vi "zmq_socket_set.vi"(7 "dll":path, 8 "error in":errorcluster, 10 "socket":u64, 11 "context":u64) -> (0 "error out":errorcluster, 3 "socket out":refnum<class "Socket.lvclass">)   [LabVIEW 2025, in "ZeroMQ.lvlib" / "Socket.lvclass"]
uses:
  Socket.lvclass
  Socket.lvclass/Socket.ctl
panel:
  # "ØMQ"
  # "labview"
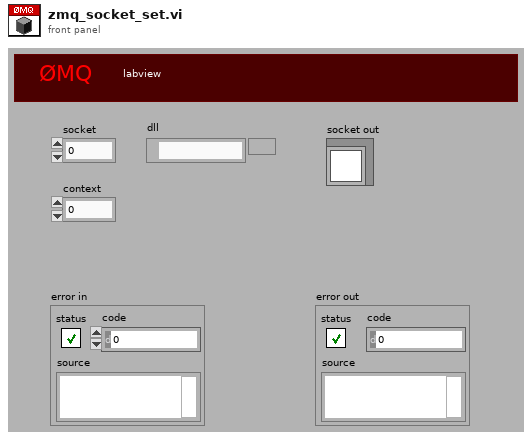
[diagram p1: front panel]
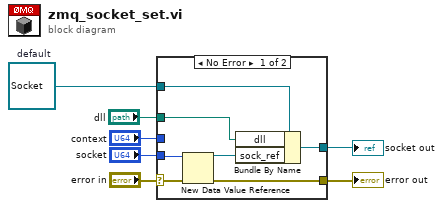
[diagram p0: block diagram]
diagram:
  w7 = refnum<class "Socket.lvclass"> refnum  # default
  n1 = case shown="No Error" "error in" {
    selector: "error in" -> [w9 w15]
    tunnel: w7 -> [w14 _]
    tunnel: [w13 _] -> w6
    tunnel: [w10 w15] -> w4
    tunnel: "context" -> [_ _]
    tunnel: "socket" -> [w11 _]
    tunnel: "dll" -> [w8 _]
    frame No Error {
      n2 = New Data Value Reference(data value=w11, error in=w9) -> (data value reference=w12:refnum<data-value>, error out=w10:errorcluster)
      n3 = Bundle By Name(cluster=w14, "dll"=w8, "sock_ref"=w12) -> (w13:refnum<class "Socket.lvclass">)
    }
    frame Error {
    }
  }
  "socket out" <- w6
  "error out" <- w4
